vi "enable_channel_ASIC_mezzanine.vi"(4 "Clip_sel_b":u32=1, 5 "maj/sum":bool, 6 "Ib_clipVb":u32=63, 7 "Att gain":u32, 8 "error in":errorcluster, 9 "Channel":u32=6, 10 "id_in":i32, 11 "connection ID":refnum<k5>) -> (0 "error out":errorcluster, 1 "id_out":i32=1, 3 "connection ID out":refnum<k5>)   [LabVIEW 2012]
doc: "This VI sends a command to the Integration Board and provides the received data when necessary."
panel:
  out "written data":u32=16063
  out "data out serial":string="Channels activated"
  out "data read value":u32=16063
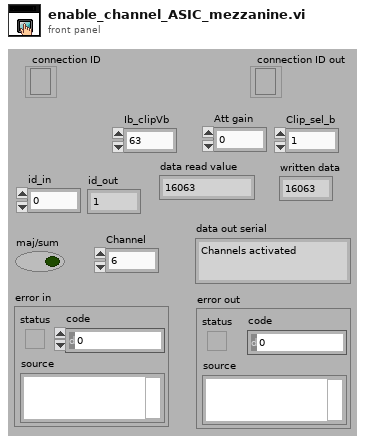
[diagram p1: front panel]
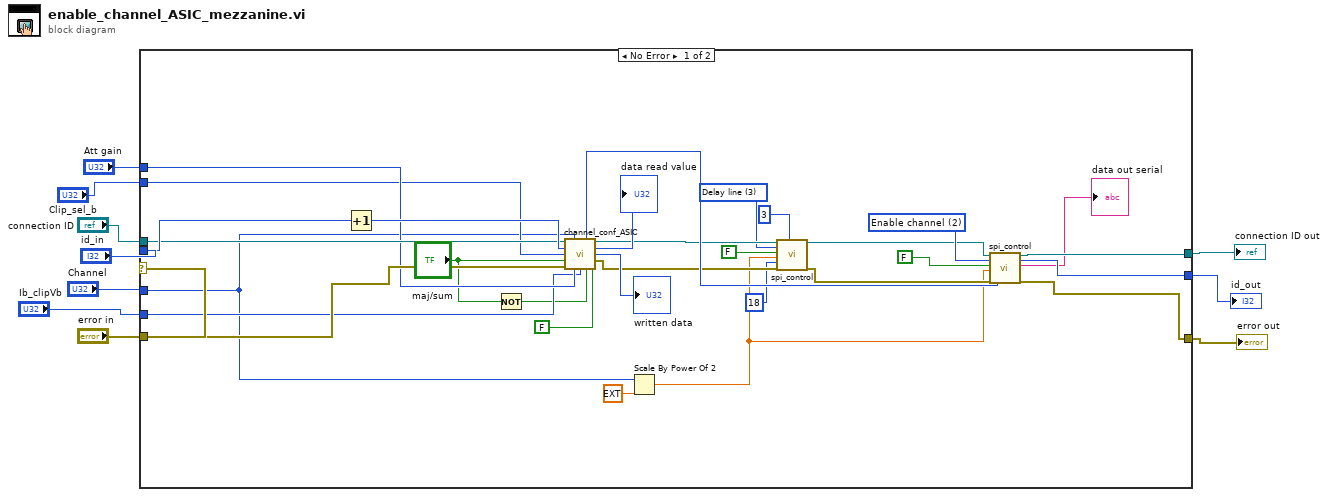
[diagram p0: block diagram]
diagram:
  n1 = case shown="No Error" "error in" {
    tunnel: "id_in" -> [w35 w41]
    tunnel: "error in" -> [w33 w42]
    tunnel: "connection ID" -> [w34 w43]
    tunnel: [w31 w42] -> w8
    tunnel: [w32 w43] -> w7
    tunnel: "Channel" -> [w25 _]
    tunnel: [w30 w41] -> w5
    tunnel: "Att gain" -> [w28 _]
    tunnel: "Ib_clipVb" -> [w27 _]
    tunnel: "Clip_sel_b" -> [w26 _]
    frame No Error {
      w15 = u16 3 items=["Attenuation", "Clipping", "Enable channel", "Delay line", "ASIC"] ("Device")
      w38 = u16 2 items=["Attenuation", "Clipping", "Enable channel", "Delay line", "ASIC"] ("Device")
      n2 = Increment(x=w35) -> (x+1=w40:i32)
      n3 = Not(x="maj/sum") -> (.not. x?=w21:bool)
      n4 = call "channel_conf_ASIC.vi"("connection ID"=w34, "Ring"=w25, "Id in"=w40, "Clip_sel_b"=w26, "CompBuf_en_b"="maj/sum", "error out"=w33, "Att gain"=w28, "Ib_ClipVb"=w27, "Clip_en_b"=w21, "Att_en_b"=FALSE) -> ("Id out"=w39:i32, "connection ID out"=w19:refnum<k5>, "data read value"=→"data read value":u32, "written data"=→"written data":u32, "error out 2"=w17:errorcluster)  [unwired: 1 in]
      n5 = Scale By Power Of 2(n=w25, x=ext 1.0) -> (x*2^n=w14:ext)
      n6 = call "spi_control.vi"("connection ID"=w19, "Device"=w15, "Read/#write"=FALSE, "Data"=w14, "Register or channel"=18, "error in"=w17, "chip delay"=3) -> ("connection ID out"=w18:refnum<k5>, "error out 2"=w16:errorcluster)  [unwired: 5 in, 6 out]
      n7 = call "spi_control.vi"("connection ID"=w18, "Device"=w38, "Read/#write"=FALSE, "Data"=w14, "error in"=w16, "Id in"=w39) -> ("connection ID out"=w32:refnum<k5>, "Id out"=w30:i32, "data out serial"=→"data out serial":string, "error out 2"=w31:errorcluster)  [unwired: 6 in, 4 out]
    }
    frame Error {
    }
  }
  "error out" <- w8
  "connection ID out" <- w7
  "id_out" <- w5
